vi "Periodic Tasks.vi"(8 "error in":errorcluster) -> ()   [LabVIEW 2011]
doc: "This VI runs in parallel to other tasks. It can contain as many user-defined periodic loops as you need. These can carry out PID or other sorts of timed response."
uses:
  <vilib>/Rock Robotics/WPI/Relay/WPI_RelayValue.ctl
  <vilib>/Rock Robotics/SystemInterfaces/Utilities/FPGA_UtilitiesLED State.ctl
  <vilib>/Rock Robotics/SystemInterfaces/Utilities/FPGA_UtilitiesLED Source.ctl
  Robot Global Data.vi
panel:
  in  "Camera Lock 2":bool
  out "Distance (ft) 2":dbl
  out "Position.Y 2":dbl
  out "Position.X 2":dbl
  in  "Target Info 2":T1(array[cluster])
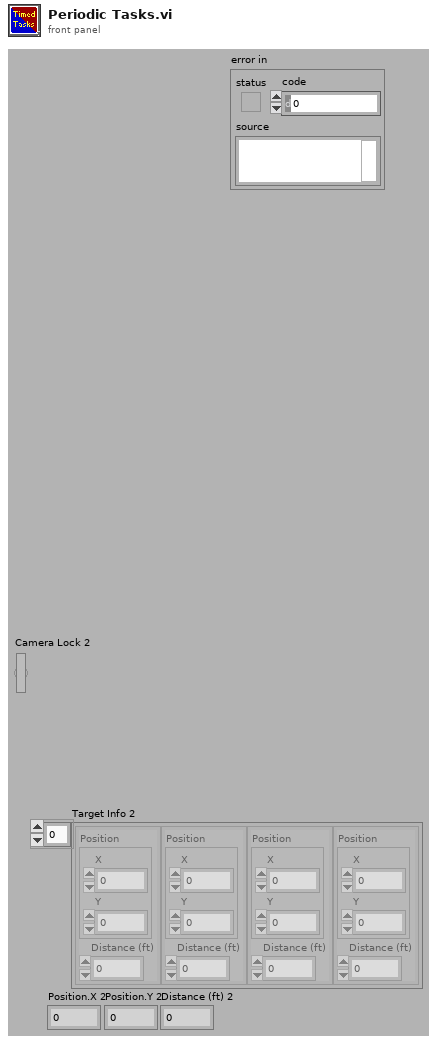
[diagram p1: front panel]
types:
  T1 = cluster{"Position":cluster{"X":dbl, "Y":dbl}, "Distance (ft)":dbl}[]
  T2 = typedef "WPI_JoystickDevRef.ctl" = cluster{"Device":T3}
  T3 = typedef "WPI_JoystickDeviceEnum.ctl" = enum16{"USB 1", "USB 2", "USB 3", "USB 4", "Kinect 1", "Kinect 2"}
  T4 = typedef "WPI_RobotDriveDevRef.ctl" = cluster{"DevStatus":errorcluster, "Motors[]":T5[], "Square Inputs":bool, "Max Output":dbl, "Isochronous":bool}
  T5 = typedef "WPI_MotorControlDeviceRef.ctl" = cluster{"DeviceStatus":errorcluster, "Type":enum16{"PWM", "CAN"}, "PWM":cluster{"Digital Module":T6, "PWM Channel":T7, "DeadBand":T8}, "CAN":cluster{"Device Number":u8, "Control Mode":T9, "Semaphore":T10, "Max Vout":dbl}, "Invert":bool, "TransformRef":T11, "InvTransformRef":T11}
  T6 = typedef "FPGA_TypedefDigitalModule.ctl" = enum16{"Digital Module 1", "Digital Module 2"}
  T7 = typedef "FPGA_DIOPWMChannel.ctl" = enum8{"PWM 1", "PWM 2", "PWM 3", "PWM 4", "PWM 5", "PWM 6", "PWM 7", "PWM 8", "PWM 9", "PWM 10", "Invalid"}
  T8 = typedef "WPI_PWMDeadband.ctl" = cluster{"Name":string, "maxPositivePwm":i32, "minPositivePwm":i32, "centerPwm":i32, "maxNegativePwm":i32, "minNegativePwm":i32, "angularRange":u16}
  T9 = typedef "WPI_CANJaguar_ControlMode.ctl" = enum8{"Percent VBus", "Current", "Speed", "Position", "Voltage"}
  T10 = typedef "Semaphore RefNum" = refnum<k1>
  T11 = typedef "WPI_PWMTransform_ConPane.ctl" = refnum<vi>
  T12 = cluster{"JoystickDevRef":T2, "RobotDriveDevRef":T4}
  T13 = typedef "WPI_EncoderDevRef.ctl" = cluster{"DevStatus":errorcluster, "EncoderIndex":T14, "CounterIndex":T15, "DistancePerCount":dbl, "Decoding Type":T16}
  T14 = typedef "FPGA_EncoderIdx.ctl" = enum8{"Enc 0", "Enc 1", "Enc 2", "Enc 3", "Invalid"}
  T15 = typedef "FPGA_CounterCtrSystemIndex.ctl" = enum8{"Ctr 0", "Ctr 1", "Ctr 2", "Ctr 3", "Ctr 4", "Ctr 5", "Ctr 6", "Ctr 7", "Invalid"}
  T16 = typedef "WPI_EncoderType.ctl" = enum16{"1x", "2x", "4x"}
  T17 = typedef "WPI_RelayValue.ctl" = enum16{"Off", "On", "Forward", "Reverse"}
  T18 = cluster{"axis 1 (x)":dbl, "axis 2 (y)":dbl, "axis 3 (throttle)":dbl, "axis 4":dbl, "axis 5":dbl, "axis 6":dbl}
  T19 = cluster{"Position":cluster{"X":dbl, "Y":dbl}, "Distance (ft)":dbl}
  T20 = typedef "WPI_RelayDevRef.ctl" = cluster{"DevStatus":errorcluster, "Relay Channel":T21, "Digital Module":T6, "Relay Direction":T22}
  T21 = typedef "FPGA_DIORelayChannel.ctl" = enum8{"Relay 1", "Relay 2", "Relay 3", "Relay 4", "Relay 5", "Relay 6", "Relay 7", "Relay 8", "Invalid"}
  T22 = typedef "WPI_RelayDirection.ctl" = enum16{"Both directions", "Forward only", "Reverse only"}
  T23 = typedef "WPI_GyroDevRef.ctl" = cluster{"DevStatus":errorcluster, "Analog Module":T24, "Analog Channel":T25, "Offset":dbl, "Gain (VoltsPerDegree/Second)":dbl}
  T24 = typedef "FPGA_TypedefAnalogModule.ctl" = enum16{"Analog Module 1", "Analog Module 2"}
  T25 = typedef "FPGA_AIChannel.ctl" = enum8{"AI 1", "AI 2", "AI 3", "AI 4", "AI 5", "AI 6", "AI 7", "AI 8", "Invalid"}
  T26 = typedef "FPGA_UtilitiesLED State.ctl" = enum16{"Off", "On", "Toggle"}
  T27 = typedef "FPGA_UtilitiesLED Source.ctl" = enum16{"User LED", "FPGA LED"}
  T28 = typedef "WPI_CompressorDevRef.ctl" = cluster{"DevStatus":errorcluster, "DigitalInputDevRef":T29, "RelayDevRef":T20}
  T29 = typedef "WPI_DigitalInputDevRef.ctl" = cluster{"DevStatus":errorcluster, "DIO Channel":T30, "Digital Module":T6}
  T30 = typedef "FPGA_DIOChannel.ctl" = enum8{"DIO 1", "DIO 2", "DIO 3", "DIO 4", "DIO 5", "DIO 6", "DIO 7", "DIO 8", "DIO 9", "DIO 10", "DIO 11", "DIO 12", "DIO 13", "DIO 14", "Invalid"}
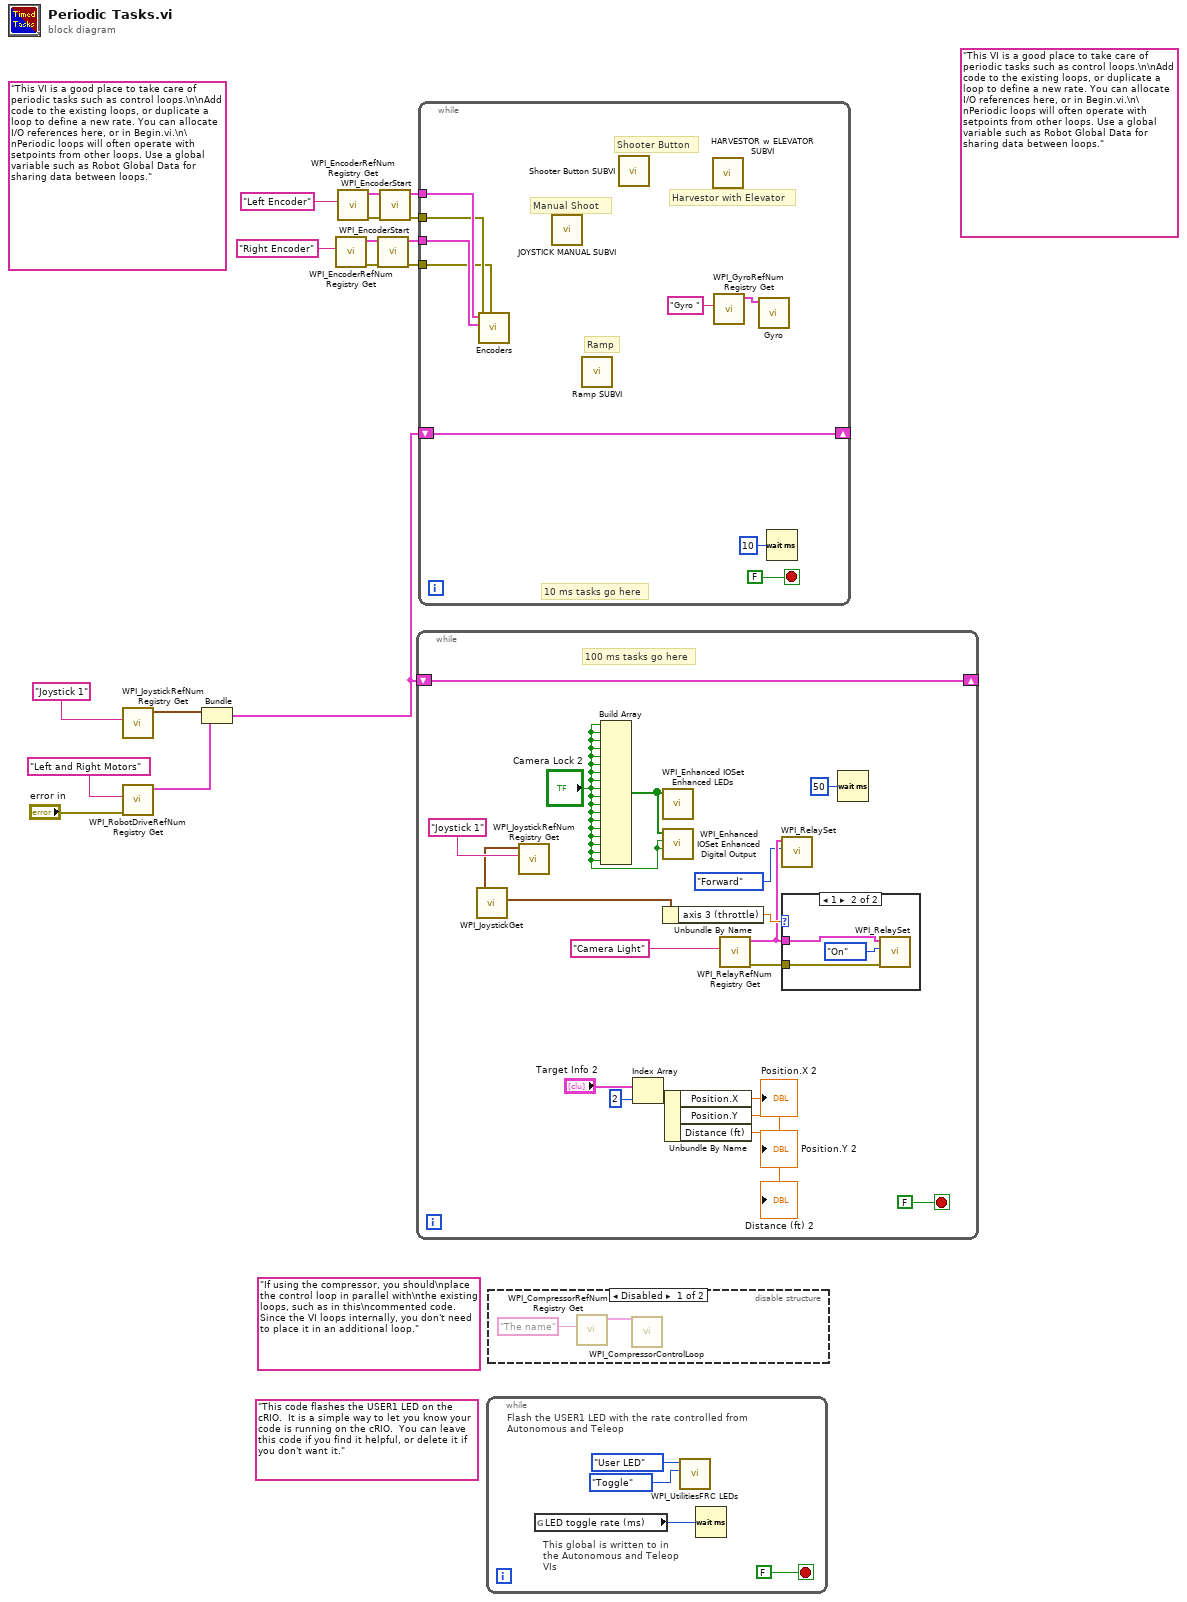
[diagram p0: block diagram]
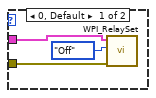
[diagram p3: hidden frame]
diagram:
  (unwired) "This VI is a good place to take care of periodic tasks such as control loops.\n\nAdd code to the existing loops, or duplicate a loop to define a new rate. You can allocate I/O references here, or in Begin.vi.\n\nPeriodic loops will often operate with setpoints from other loops. Use a global variable such as Robot Global Data for sharing data between loops."
  (unwired) "If using the compressor, you should\nplace the control loop in parallel with\nthe existing loops, such as in this\ncommented code. Since the VI loops internally, you don't need to place it in an additional loop."
  (unwired) "This code flashes the USER1 LED on the cRIO.  It is a simple way to let you know your code is running on the cRIO.  You can leave this code if you find it helpful, or delete it if you don't want it."
  (unwired) "This VI is a good place to take care of periodic tasks such as control loops.\n\nAdd code to the existing loops, or duplicate a loop to define a new rate. You can allocate I/O references here, or in Begin.vi.\n\nPeriodic loops will often operate with setpoints from other loops. Use a global variable such as Robot Global Data for sharing data between loops."
  n1 = call <vilib>:"WPI_JoystickRefNum Registry Get.vi"("refnum name"="Joystick 1") -> ("JoystickDevRef"=w1:T2)  [unwired: 1 in, 9 out]
  n2 = call <vilib>:"WPI_RobotDriveRefNum Registry Get.vi"("error in (no error)"="error in", "refnum name"="Left and Right Motors") -> ("RobotDriveDevRef"=w14:T4)  [unwired: 9 out]
  n3 = Bundle("JoystickDevRef"=w1, "RobotDriveDevRef"=w14) -> (w13:T12)  [unwired: 1 out]
  n4 = call <vilib>:"WPI_EncoderRefNum Registry Get.vi"("refnum name"="Right Encoder") -> ("error out"=w8:errorcluster, "EncoderDevRef"=w9:T13)  [unwired: 9 in]
  n5 = call <vilib>:"WPI_EncoderRefNum Registry Get.vi"("refnum name"="Left Encoder") -> ("error out"=w6:errorcluster, "EncoderDevRef"=w7:T13)  [unwired: 9 in]
  n6 = call <vilib>:"WPI_EncoderStart.vi"("error in (no error)"=w8, "EncoderDevRef"=w9) -> ("error out"=w2:errorcluster, "EncoderDevRef"=w4:T13)  [unwired: 8 in]
  n7 = call <vilib>:"WPI_EncoderStart.vi"("error in (no error)"=w6, "EncoderDevRef"=w7) -> ("error out"=w3:errorcluster, "EncoderDevRef"=w5:T13)  [unwired: 8 in]
  n8 = while {
    shift-right: [w33] -> _
    shift-left: w13 -> [w33]
    stop <- FALSE stop-if-true
    # "100 ms tasks go here"
    n9 = call <vilib>:"WPI_JoystickRefNum Registry Get.vi"("refnum name"="Joystick 1") -> ("JoystickDevRef"=w17:T2)  [unwired: 1 in, 9 out]
    n10 = call <vilib>:"WPI_JoystickGet.vi"("JoystickDevRef"=w17) -> ("Axes"=w19:T18)  [unwired: 4 in, 2 out]
    n11 = Build Array("Camera Lock 2", "Camera Lock 2", "Camera Lock 2", "Camera Lock 2", "Camera Lock 2", "Camera Lock 2", "Camera Lock 2", "Camera Lock 2", "Camera Lock 2", "Camera Lock 2", "Camera Lock 2", "Camera Lock 2", "Camera Lock 2", "Camera Lock 2", "Camera Lock 2", "Camera Lock 2", "Camera Lock 2", "Camera Lock 2") -> (w20:bool[])
    n12 = Index Array(array="Target Info 2", index=2) -> (element=w30:T19)
    n13 = call <vilib>:"WPI_Enhanced IOSet Enhanced LEDs.vi"("LEDs [1-8]"=w20) -> ()  [unwired: 10 in, 1 out]
    n14 = call <vilib>:"WPI_Enhanced IOSet Enhanced Digital Output.vi"("Digital Output HC2"="Camera Lock 2", "Digital Output HC1"="Camera Lock 2", "Digital Output [1-16]"=w20) -> ()  [unwired: 8 in, 1 out]
    n15 = Unbundle By Name(w19) -> ("axis 3 (throttle)"=w24:dbl)
    n16 = Unbundle By Name(w30) -> ("Position.X"=→"Position.X 2":dbl, "Position.Y"=→"Position.Y 2":dbl, "Distance (ft)"=→"Distance (ft) 2":dbl)
    n17 = call <vilib>:"WPI_RelayRefNum Registry Get.vi"("refnum name"="Camera Light") -> ("error out"=w25:errorcluster, "RelayDevRef"=w23:T20)  [unwired: 9 in]
    n18 = call <vilib>:"WPI_RelaySet.vi"("RelayValue"=WPI_RelayValue."Forward", "RelayDevRef"=w23) -> ()  [unwired: 8 in, 2 out]
    n19 = case shown="1" w24 {
      tunnel: w23 -> [w38 w41]
      tunnel: w25 -> [w37 w40]
      frame 0, Default {
        n20 = call <vilib>:"WPI_RelaySet.vi"("error in (no error)"=w37, "RelayValue"=WPI_RelayValue."Off", "RelayDevRef"=w38) -> ()  [unwired: 7 in, 2 out]
      }
      frame 1 {
        n21 = call <vilib>:"WPI_RelaySet.vi"("error in (no error)"=w40, "RelayValue"=WPI_RelayValue."On", "RelayDevRef"=w41) -> ()  [unwired: 7 in, 2 out]
      }
    }
    n22 = Wait (ms)(milliseconds to wait=u32 50) -> ()  [unwired: 1 out]
  }
  n23 = while {
    shift-right: [w48] -> _
    shift-left: w13 -> [w48]
    tunnel: w5 -> [w47]
    tunnel: w4 -> [w46]
    tunnel: w3 -> [w45]
    tunnel: w2 -> [w44]
    stop <- FALSE stop-if-true
    # "Manual Shoot"
    # "Harvestor with Elevator"
    # "Shooter Button"
    # "Ramp"
    # "10 ms tasks go here"
    n24 = call "Encoders.vi"("error in (no error) 2"=w44, "error in (no error)"=w45, "Left Encoder"=w46, "Right Encoder"=w47) -> ()  [unwired: 8 out]
    n25 = call "JOYSTICK MANUAL SUBVI.vi"() -> ()  [unwired: 12 in]
    n26 = call "Ramp SUBVI.vi"() -> ()  [unwired: 12 in]
    n27 = call "Shooter Button SUBVI.vi"() -> ()  [unwired: 12 in]
    n28 = call "HARVESTOR w ELEVATOR  SUBVI.vi"() -> ()  [unwired: 12 in]
    n29 = call <vilib>:"WPI_GyroRefNum Registry Get.vi"("Gyro"="Gyro " ("refnum name")) -> ("GyroDevRef"=w42:T23)  [unwired: 1 in, 9 out]
    n30 = call "Gyro.vi"("GyroDevRef"=w42) -> ()  [unwired: 1 in, 10 out]
    n31 = Wait (ms)(milliseconds to wait=u32 10) -> ()  [unwired: 1 out]
  }
  n32 = while {
    stop <- FALSE stop-if-true
    # "This global is written to in the Autonomous and Teleop VIs"
    # "Flash the USER1 LED with the rate controlled from Autonomous and Teleop"
    n33 = global read "Robot Global Data.vi" "LED toggle rate (ms)"() -> (w51:u32)
    n34 = call <vilib>:"WPI_UtilitiesFRC LEDs.vi"("State"=FPGA_UtilitiesLED_State."Toggle", "LED Type"=FPGA_UtilitiesLED_Source."User LED") -> ()  [unwired: 1 in, 9 out]
    n35 = Wait (ms)(milliseconds to wait=w51) -> ()  [unwired: 1 out]
  }
  n36 = disable-structure shown="Disabled" {
    frame Disabled {
      n37 = call <vilib>:"WPI_CompressorRefNum Registry Get.vi"("refnum name"="The name") -> ("CompressorDevRef"=w56:T28)  [unwired: 9 in, 1 out]
      n38 = call <vilib>:"WPI_CompressorControlLoop.vi"("CompressorDevRef"=w56) -> ()  [unwired: 11 in]
    }
    frame Enabled {
    }
  }
